vi "Msg Display.vi"(6 "ShowIgnoreBtn":bool, 7 "ManTaskQ Ref":refnum<queue>, 9 "Btn Txt":enum16{"OK/Cancel", "YES/NO", "OK"}(ring), 10 "Msg Display":string caption="String", 11 "PowerSupply":bool) -> (2 "Ignore Out":bool, 3 "OK Out":bool)   [LabVIEW 2024]
uses:
  MFActor/MainFormTaskName.ctl
  Global Variables.vi
panel:
  in  "Ignore Button":bool
  in  "Power Supply":T1={"Voltage"=1.0, "Current"=0.0, "Frequency"=45.0, "Time"=0.0} caption="電源供應器" {"Frequency" min=0.0 max=1000.0 format="%#_6f"; "Time" min=0.0 max=10.0; "Voltage" min=0.0 max=500.0}
  in  "POwer OFF":bool
  in  "Power ON":bool
  in  "Cancel Button":bool
  in  "OK Button":bool
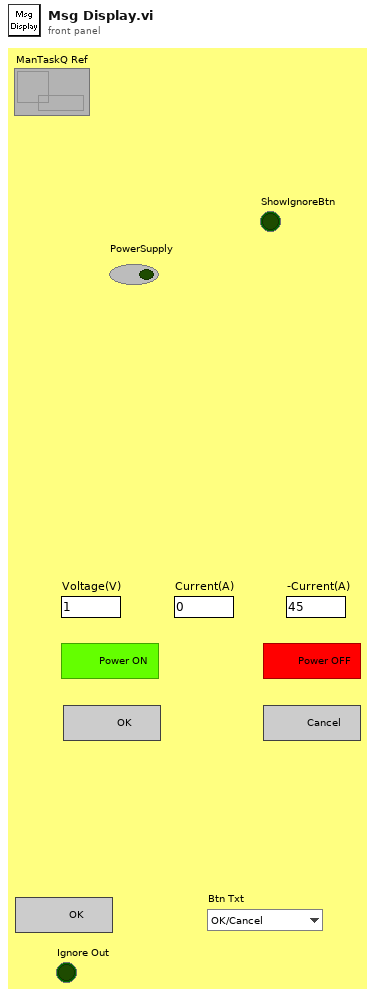
[diagram p1: front panel]
types:
  T1 = cluster{"Voltage":dbl, "Current":dbl, "Frequency":dbl, "Time":dbl}
  T2 = typedef "MainFormTaskName.ctl" = enum16{"None", "InitMainForUI", "InitInterfaceCards", "OpenDIOCard", "CloseDIOCard", "OpenAIOCard", "CloseAIOCard", "OpenRED", "CloseRED", "Open4503B", "Close4503B", "OpenPW3390", "ClosePW3390", "Open4118", "Close4118", "OpenPID", "ClosePID", "OpenRmtService", "CloseRmtService", "QueryData", "ZeroAngle", "ErrCodeHandler", "RestError", "DIHandler", "SendDO", "SendAO", "LoadRecipe", "RefreshPIDUI", "WriteRecipe", "EditMultiPt", "LoadSetting", "WriteSetting", "InitDev", "CloseDev", "SetDriverTQ", "SetTorque", "DriveSinTQ", "SinTorque", "SetSpeed", "ActiveMotor", "RunPID", "StartRunPIDAdj", "InitAutoUI", "RefreshAutoUI", "LeaveAutoTestUI", "UpdateRecipeContent", "StartTestProc", "StopTestProc", "CleanTestData", "InitCalibration", "LeaveCalibration", "Calibration", "SelectExportedFileType", "ExportAsCSV", "ExportAsXls", "SoftwareReady", "ShowPSMsg", "DCPowerCtrl", "ExitApp"}
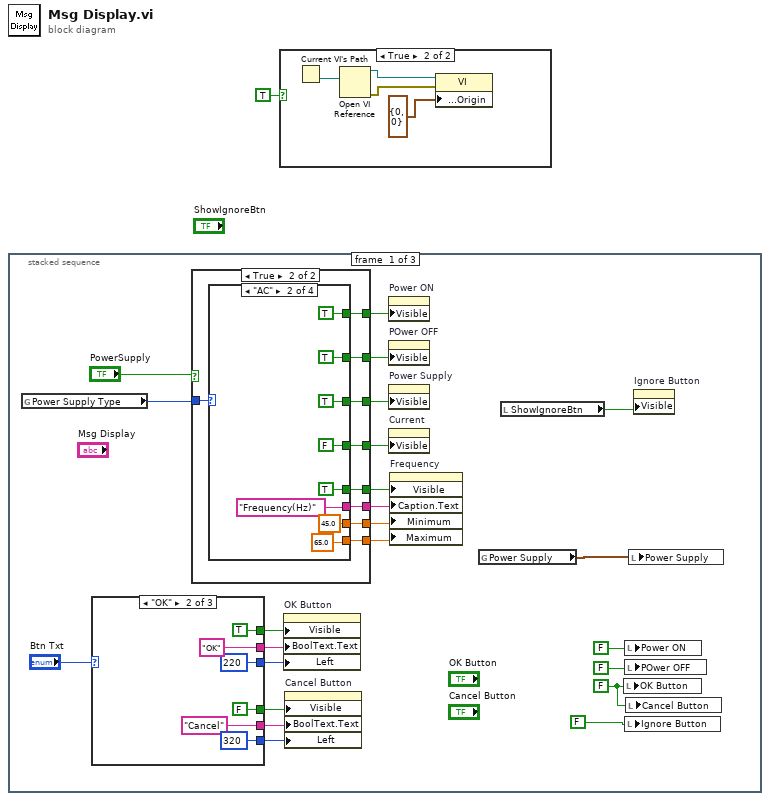
[diagram p0: block diagram]
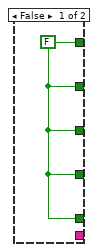
[diagram p3: hidden frame]
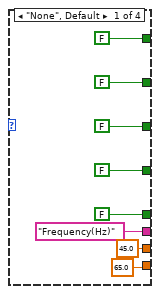
[diagram p4: hidden frame]
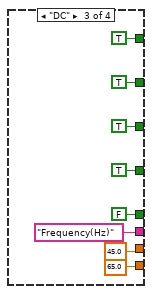
[diagram p5: hidden frame]
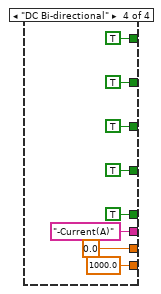
[diagram p6: hidden frame]
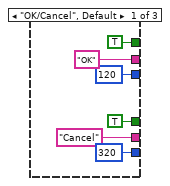
[diagram p7: hidden frame]
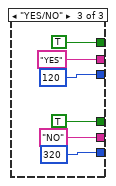
[diagram p8: hidden frame]
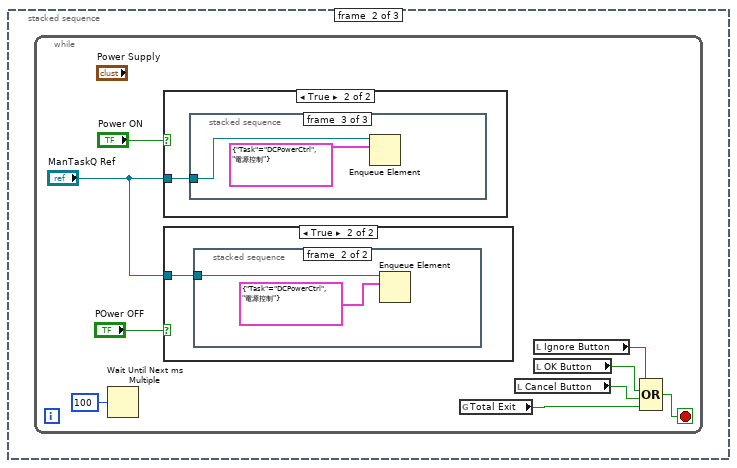
[diagram p9: hidden frame]
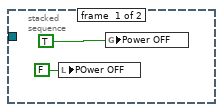
[diagram p11: hidden frame]
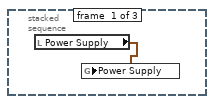
[diagram p13: hidden frame]
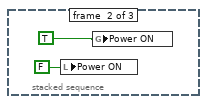
[diagram p14: hidden frame]
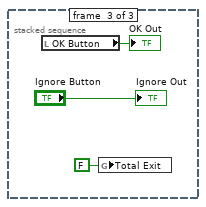
[diagram p15: hidden frame]
diagram:
  n1 = stacked-sequence {
    frame #0 {
      w24 = FALSE ("OK Button")
      n2 = global read "Global Variables.vi" "Power Supply Type"() -> (w3:enum16{"None", "AC", "DC", "DC Bi-directional"})
      n3 = case shown="\"OK\"" "Btn Txt" {
        tunnel: ["OK" ("Boolean Text.Text") "OK" ("Boolean Text.Text") "YES" ("Boolean Text.Text")] -> w22
        tunnel: ["Cancel" ("Boolean Text.Text") "Cancel" ("Boolean Text.Text") "NO" ("Boolean Text.Text")] -> w21
        tunnel: [TRUE ("Visible") TRUE ("Visible") TRUE ("Visible")] -> w7
        tunnel: [120 ("Position:Left") 220 ("Position:Left") 120 ("Position:Left")] -> w6
        tunnel: [TRUE ("Visible") FALSE ("Visible") TRUE ("Visible")] -> w5
        tunnel: [320 ("Position:Left") 320 ("Position:Left") 320 ("Position:Left")] -> w4
        frame "OK/Cancel", Default {
        }
        frame "OK" {
        }
        frame "YES/NO" {
        }
      }
      n4 = case shown="True" "PowerSupply" {
        tunnel: w3 -> [_ w34]
        tunnel: [w25 w33] -> w18
        tunnel: [w25 w32] -> w17
        tunnel: [w25 w31] -> w16
        tunnel: [w25 w30] -> w15
        tunnel: [w25 w29] -> w14
        tunnel: [_ w28] -> w13
        tunnel: [_ w27] -> w12
        tunnel: [_ w26] -> w11
        frame False {
          w25 = FALSE
        }
        frame True {
          n5 = case shown="\"AC\"" w34 {
            tunnel: [FALSE TRUE TRUE TRUE] -> w33
            tunnel: [FALSE TRUE FALSE TRUE] -> w32
            tunnel: [FALSE FALSE TRUE TRUE] -> w31
            tunnel: [FALSE TRUE TRUE TRUE] -> w30
            tunnel: [FALSE TRUE TRUE TRUE] -> w29
            tunnel: ["Frequency(Hz)" ("Caption.Text") "Frequency(Hz)" ("Caption.Text") "Frequency(Hz)" ("Caption.Text") "-Current(A)" ("Caption.Text")] -> w28
            tunnel: [45.0 45.0 45.0 0.0] -> w27
            tunnel: [65.0 65.0 65.0 1000.0] -> w26
            frame "None", Default {
            }
            frame "AC" {
            }
            frame "DC" {
            }
            frame "DC Bi-directional" {
            }
          }
        }
      }
      n6 = property on="OK Button" class="Bool (strict)"("Visible"=w7, "BoolText.Text"=w22, "Left"=w6) -> ()  [unwired: 2 in, 2 out]
      n7 = property on="Cancel Button" class="Bool (strict)"("Visible"=w5, "BoolText.Text"=w21, "Left"=w4) -> ()  [unwired: 2 in, 2 out]
      n8 = property on="Power ON" class="Bool (strict)"("Visible"=w18) -> ()  [unwired: 2 in, 2 out]
      n9 = property on="POwer OFF" class="Bool (strict)"("Visible"=w14) -> ()  [unwired: 2 in, 2 out]
      n10 = property on="Power Supply" class="Clust (strict)"("Visible"=w15) -> ()  [unwired: 2 in, 2 out]
      n11 = property on="Current" class="DigNum (strict)"("Visible"=w16) -> ()  [unwired: 2 in, 2 out]
      n12 = property on="Frequency" class="DigNum (strict)"("Visible"=w17, "Caption.Text"=w13, "Minimum"=w12, "Maximum"=w11) -> ()  [unwired: 2 in, 2 out]
      n13 = global read "Global Variables.vi" "Power Supply"() -> (w2:T1)
      n14 = local read "ShowIgnoreBtn"() -> (w9:bool)
      n15 = local write "OK Button"(w24) -> ()
      n16 = local write "Power ON"(FALSE ("Power ON")) -> ()
      n17 = local write "POwer OFF"(FALSE ("Power ON")) -> ()
      n18 = local write "Ignore Button"(FALSE) -> ()
      n19 = local write "Cancel Button"(w24) -> ()
      n20 = local write "Power Supply"(w2) -> ()
      n21 = property on="Ignore Button" class="Bool (strict)"("Visible"=w9) -> ()  [unwired: 2 in, 2 out]
    }
    frame #1 {
      n22 = while {
        stop <- w92 stop-if-true
        n23 = Wait Until Next ms Multiple(millisecond multiple=u32 100) -> ()  [unwired: 1 out]
        n24 = case shown="True" "Power ON" {
          tunnel: "ManTaskQ Ref" -> [_ w99]
          frame False {
          }
          frame True {
            n25 = stacked-sequence {
              tunnel: w99 -> [_ _ w104]
              frame #0 {
                n26 = local read "Power Supply"() -> (w100:T1)
                n27 = global write "Global Variables.vi" "Power Supply"(w100) -> ()
              }
              frame #1 {
                n28 = local write "Power ON"(FALSE ("Power ON")) -> ()
                n29 = global write "Global Variables.vi" "Power ON"(TRUE ("Total Exit")) -> ()
              }
              frame #2 {
                n30 = Enqueue Element(queue=w104, element=cluster{"Task":T2, string} {"Task"=enum."DCPowerCtrl", "電源控制"}) -> ()  [unwired: 2 in, 3 out]
              }
            }
          }
        }
        n31 = case shown="True" "POwer OFF" {
          tunnel: "ManTaskQ Ref" -> [_ w94]
          frame False {
          }
          frame True {
            n32 = stacked-sequence {
              tunnel: w94 -> [_ w98]
              frame #0 {
                n33 = local write "POwer OFF"(FALSE ("Power ON")) -> ()
                n34 = global write "Global Variables.vi" "Power OFF"(TRUE ("Total Exit")) -> ()
              }
              frame #1 {
                n35 = Enqueue Element(queue=w98, element=cluster{"Task":T2, string} {"Task"=enum."DCPowerCtrl", "電源控制"}) -> ()  [unwired: 2 in, 3 out]
              }
            }
          }
        }
        n36 = global read "Global Variables.vi" "Total Exit"() -> (w86:bool)
        n37 = local read "Cancel Button"() -> (w91:bool)
        n38 = local read "Ignore Button"() -> (w87:bool)
        n39 = local read "OK Button"() -> (w90:bool)
        n40 = Compound Arithmetic op=OR(w87, w90, w91, w86) -> (w92:bool)
      }
    }
    frame #2 {
      n41 = local read "OK Button"() -> (→"OK Out":bool)
      n42 = global write "Global Variables.vi" "Total Exit"(FALSE ("Total Exit")) -> ()
      "Ignore Out" <- "Ignore Button"
    }
  }
  n43 = case shown="True" TRUE {
    frame False {
    }
    frame True {
      n44 = Current VI's Path() -> (path=w111:path)
      n45 = Open VI Reference(vi path=w111) -> (vi reference=w110:refnum<vi>, error out=w109:errorcluster)  [unwired: 5 in]
      n46 = property class="VI"(reference=w110, error in=w109, "Front Panel Window:Origin"=cluster{"Horizontal":i16, "Vertical":i16} {"Horizontal"=0, "Vertical"=0}) -> ()  [unwired: 2 out]
    }
  }
